vi "Flip States.vi"(8 "error in":errorcluster, 11 "Context in":refnum<class "Context.lvclass">) -> (0 "error out":errorcluster, 3 "Context out":refnum<class "Context.lvclass">)   [LabVIEW 2021, in "Context.lvlib" / "Context.lvclass"]
uses:
  Context.lvclass
  C:/PPLs/Design-Patterns/State Pattern/State Pattern/State Pattern/State Pattern.lvclass
  A State/A State.lvclass
  C:/PPLs/Design-Patterns/State Pattern/Example/Context/State/State.lvclass
  Context.lvclass/Context.ctl
  B State/B State.lvclass
  State/State.lvclass
  State Pattern/State Pattern/State Pattern.lvclass
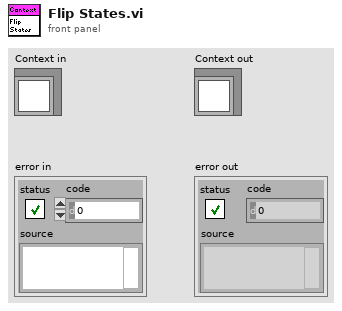
[diagram p1: front panel]
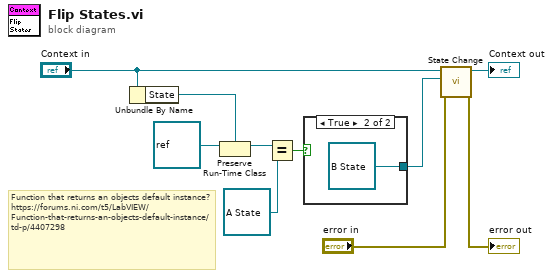
[diagram p0: block diagram]
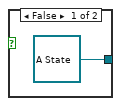
[diagram p2: hidden frame]
diagram:
  # "Function that returns an objects default instance?\nhttps://forums.ni.com/t5/LabVIEW/Function-that-returns-an-objects-default-instance/td-p/4407298"
  n1 = Unbundle By Name("Context in") -> ("State"=w9:refnum<class "State.lvclass">)
  n2 = Preserve Run-Time Class(object in=refnum<class> refnum ("LabVIEW Object"), 2:w9) -> (object out=w8:refnum<class "State.lvclass">)  [unwired: 1 in, 1 out]
  n3 = Equal?(x=w8, y=refnum<class "A State.lvclass"> refnum ("Context.lvlib:A Context State.lvclass")) -> (x = y?=w6:bool)
  n4 = case shown="True" w6 {
    tunnel: [refnum<class "A State.lvclass"> refnum ("Context.lvlib:A Context State.lvclass") refnum<class "B State.lvclass"> refnum ("Context.lvlib:B Context State.lvclass")] -> w5
    frame False {
    }
    frame True {
    }
  }
  n5 = call "State Change.vi"("error in"="error in", "Transition State"=w5, "Context in"="Context in") -> ("error out"=→"error out":errorcluster, "Context out"=→"Context out":refnum<class "Context.lvclass">)  [unwired: 7 in]
